vi "swerveImmForAuto.vi"(8 "scalespeed":dbl, 9 "x2":dbl, 10 "y1":dbl, 11 "x1":dbl) -> ()   [LabVIEW 2020]
uses:
  <vilib>/Rock Robotics/WPI/ThirdParty/Sensors/navX/_TypeDefs/FRIC_navX_DeviceNumbersTypeDef.ctl
  <vilib>/Rock Robotics/WPI/ThirdParty/REV Robotics/REVLib/Typedef/Spark MAX Control Type.ctl
  <vilib>/Rock Robotics/WPI/ThirdParty/Phoenix-LabVIEW/CANCoder/Get/CTRE_Phoenix_CANcoder_GetSensorData.vi
  <vilib>/addons/control/pid/pid.llb/PID (DBL).vi
  <vilib>/addons/control/pid/NI_PID_pid.lvlib
panel:
  in  "dt (s)":dbl=-1.0 format="%.3f"
  in  "PID gains 2":T1={"proportional gain (Kc)"=0.004667, "integral time (Ti, min)"=0.0, "derivative time (Td, min)"=0.0} {"derivative time (Td, min)" format="%.10f"; "integral time (Ti, min)" format="%.10f"; "proportional gain (Kc)" format="%.10f"}
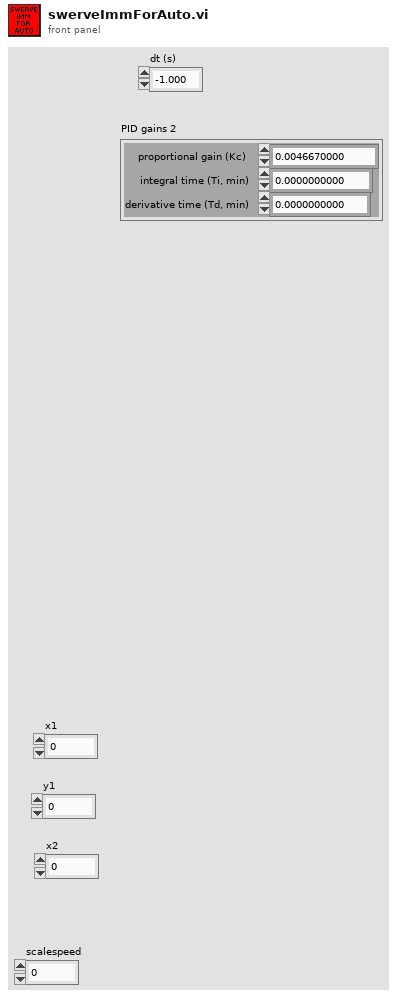
[diagram p1: front panel]
types:
  T1 = cluster{"proportional gain (Kc)":dbl, "integral time (Ti, min)":dbl, "derivative time (Td, min)":dbl}
  T2 = typedef "Spark MAX Control Type.ctl" = enum16{"Percent VBus", "Voltage", "Velocity", "Position", "Smart Motion", "Current", "Smart Velocity"}
  T3 = typedef "FRIC_navX_DeviceNumbersTypeDef.ctl" = enum16{"Dev0", "Dev1", "Dev2", "Dev3"}
  T4 = cluster{"Yaw":dbl, "Roll":dbl, "Pitch":dbl, "Heading":dbl, "Fused Heading":dbl}
  T5 = typedef "CTRE_Phoenix_CANcoder_DeviceRef.ctl" = cluster{"DeviceStatus":errorcluster, "Device Number":u8, "Handle":u64, "UsageFrame":u32, "Library Path":path}
  T6 = typedef "WPI_MotorControlDeviceRef.ctl" = cluster{"DeviceStatus":errorcluster, "Type":T7, "PWM":cluster{"PWM Channel":T8, "DeadBand":T9}, "CAN":cluster{"Device Number":u8, "SetOutput VI Ref":variant, "GetOutput VI Ref":variant, "Enable VI Ref":variant, "Disable VI Ref":variant, "Data":variant}, "Invert":bool, "DIO PWM":cluster{"PWM \"Enable\" Channel":T8, "DIOChannel":T10, "PWM Rate":dbl}}
  T7 = typedef "WPI_MotorControlType.ctl" = enum16{"PWM", "CAN", "DIO PWM"}
  T8 = typedef "FPGA_DIOPWMChannel.ctl" = enum8{"PWM 0", "PWM 1", "PWM 2", "PWM 3", "PWM 4", "PWM 5", "PWM 6", "PWM 7", "PWM 8", "PWM 9", "PWM MXP 0", "PWM MXP 1", "PWM MXP 2", "PWM MXP 3", "PWM MXP 4", "PWM MXP 5", "PWM MXP 6", "PWM MXP 7", "PWM MXP 8", "PWM MXP 9", "Invalid"}
  T9 = typedef "WPI_PWMDeadband.ctl" = cluster{"Name":string, "maxPositivePwm":i32, "minPositivePwm":i32, "centerPwm":i32, "maxNegativePwm":i32, "minNegativePwm":i32, "angularRange":u16}
  T10 = typedef "FPGA_DIOChannel.ctl" = enum8{"DIO 0", "DIO 1", "DIO 2", "DIO 3", "DIO 4", "DIO 5", "DIO 6", "DIO 7", "DIO 8", "DIO 9", "DIO MXP 0", "DIO MXP 1", "DIO MXP 2", "DIO MXP 3", "DIO MXP 4", "DIO MXP 5", "DIO MXP 6", "DIO MXP 7", "DIO MXP 8", "DIO MXP 9", "DIO MXP 10", "DIO MXP 11", "DIO MXP 12", "DIO MXP 13", "DIO MXP 14", "DIO MXP 15", "SPI Port CS1", "SPI Port CS2", "SPI Port CS3", "SPI Port MISO", "SPI Port MOSI", "Invalid"}
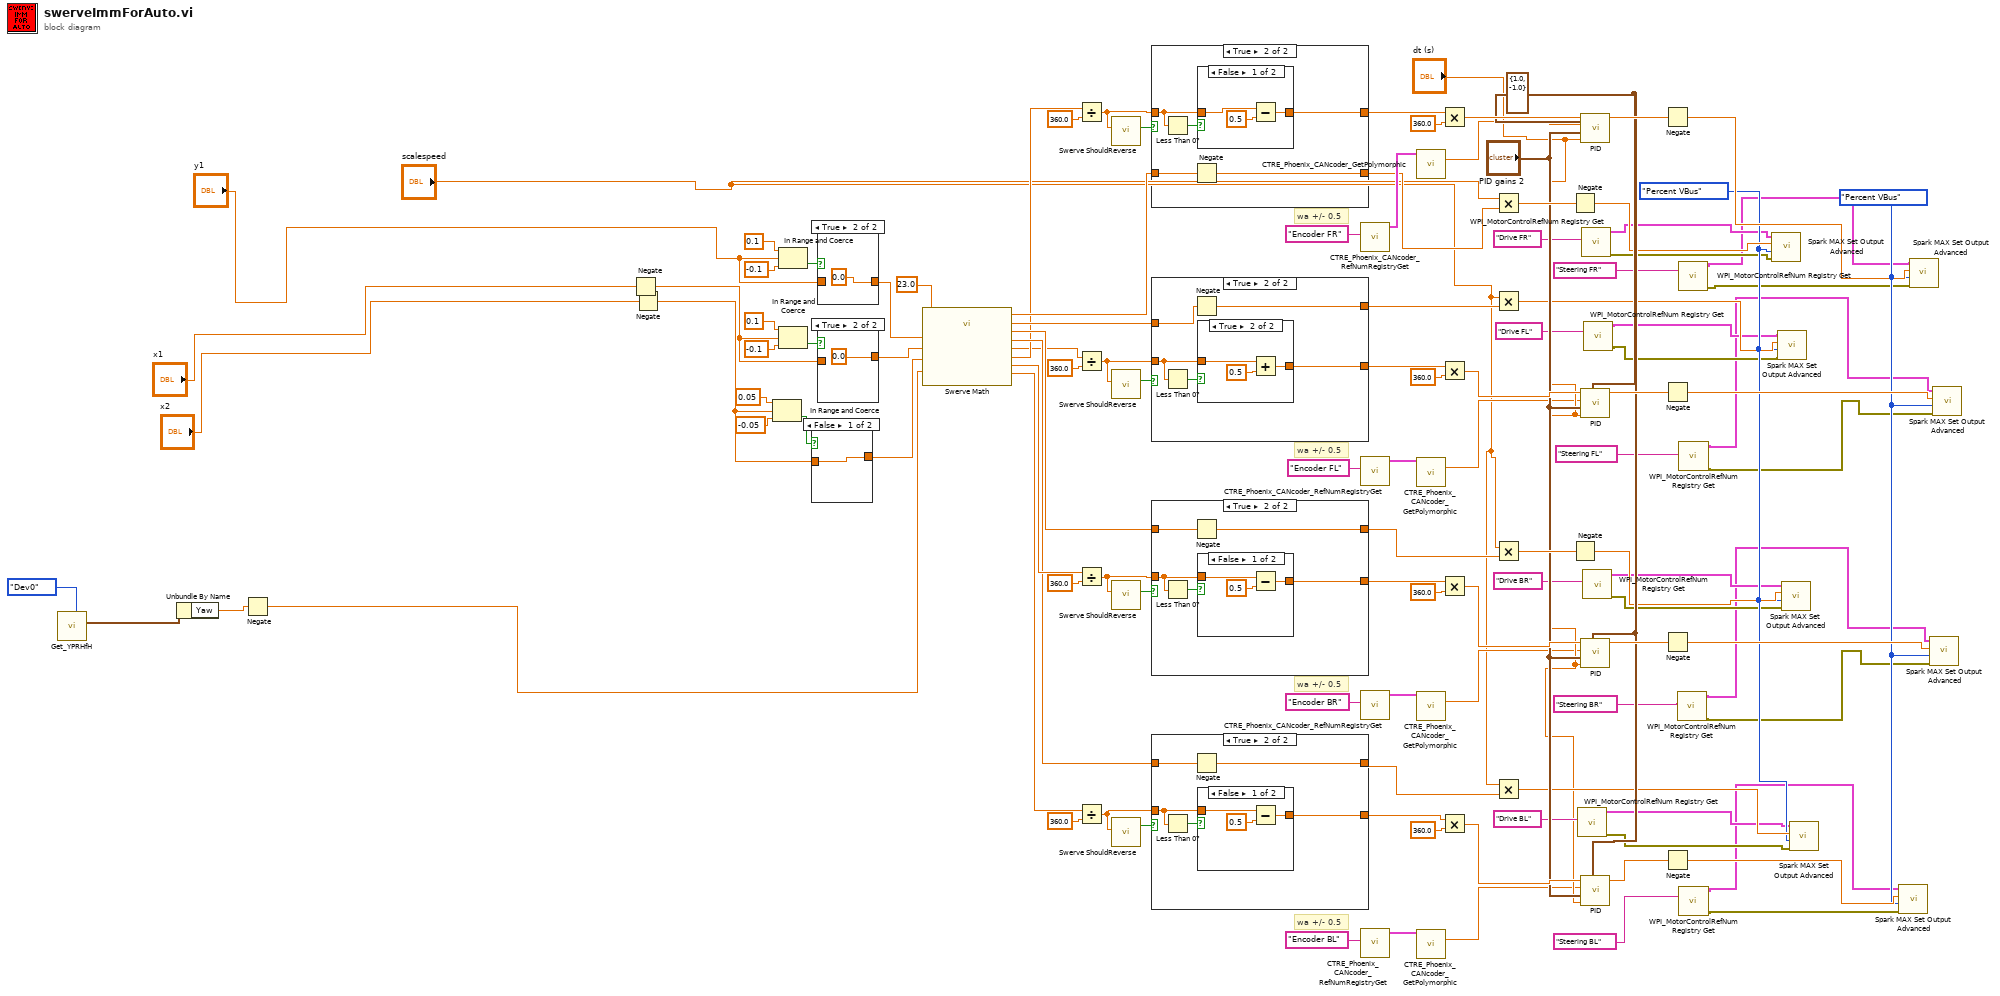
[diagram p0: block diagram]
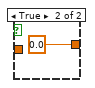
[diagram p2: hidden frame]
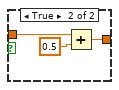
[diagram p4: hidden frame]
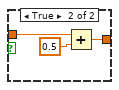
[diagram p6: hidden frame]
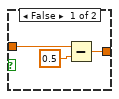
[diagram p8: hidden frame]
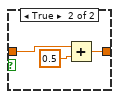
[diagram p10: hidden frame]
diagram:
  w43 = Spark_MAX_Control_Type."Percent VBus" ("Control Mode")
  w48 = Spark_MAX_Control_Type."Percent VBus" ("Control Mode")
  w53 = cluster{"output high":dbl, "output low":dbl} {"output high"=1.0, "output low"=-1.0} ("output range")
  w111 = 23.0 ("Trackwidth (W)")
  (unwired) FRIC_navX_DeviceNumbersTypeDef."Dev0" ("Device Number")
  # "wa +/- 0.5"
  # "wa +/- 0.5"
  # "wa +/- 0.5"
  # "wa +/- 0.5"
  n1 = call <vilib>:"Get_YPRHfH.vi"("Device Number"=FRIC_navX_DeviceNumbersTypeDef."Dev0") -> ("YRPHfH"=w113:T4)  [unwired: 10 in]
  n2 = Unbundle By Name(w113) -> ("Yaw"=w112:dbl)
  n3 = Negate(x=w112) -> (-x=w2:dbl)
  n4 = Negate(x="x1") -> (-x=w13:dbl)
  n5 = Negate(x="x2") -> (-x=w1:dbl)
  n6 = In Range and Coerce(upper limit=0.05, x=w1, lower limit=-0.05) -> (In Range?=w6:bool)  [unwired: 1 out]
  n7 = In Range and Coerce(upper limit=0.1, x="y1", lower limit=-0.1) -> (In Range?=w105:bool)  [unwired: 1 out]
  n8 = In Range and Coerce(upper limit=0.1, x=w13, lower limit=-0.1) -> (In Range?=w104:bool)  [unwired: 1 out]
  n9 = case shown="False" w6 {
    tunnel: [w115 0.0 ("upper limit")] -> w3
    tunnel: w1 -> [w115 _]
    frame False {
    }
    frame True {
    }
  }
  n10 = case shown="True" w105 {
    tunnel: [w117 0.0 ("upper limit")] -> w100
    tunnel: "y1" -> [w117 _]
    frame False {
    }
    frame True {
    }
  }
  n11 = case shown="True" w104 {
    tunnel: [w119 0.0 ("upper limit")] -> w101
    tunnel: w13 -> [w119 _]
    frame False {
    }
    frame True {
    }
  }
  n12 = call "Swerve Math.vi"("Trackwidth (W)"=w111, "Wheelbase (L)"=w111, "Y -FWD"=w100, "X1 STR"=w101, "X2 RCW"=w3, "Gyro Angle in degrees"=w2) -> ("wa3"=w57:dbl, "wa4"=w55:dbl, "ws1"=w60:dbl, "ws2"=w59:dbl, "ws3"=w58:dbl, "ws4"=w56:dbl, "wa2"=w12:dbl, "wa1"=w11:dbl)  [unwired: 2 in]
  n13 = Divide(x=w12, y=360.0) -> (x/y=w97:dbl)
  n14 = Divide(x=w11, y=360.0) -> (x/y=w86:dbl)
  n15 = Divide(x=w57, y=360.0) -> (x/y=w76:dbl)
  n16 = Divide(x=w55, y=360.0) -> (x/y=w65:dbl)
  n17 = call "Swerve ShouldReverse.vi"("wa in"=w97) -> ("shouldReverse out"=w98:bool)  [unwired: 10 in]
  n18 = call "Swerve ShouldReverse.vi"("wa in"=w86) -> ("shouldReverse out"=w87:bool)  [unwired: 10 in]
  n19 = call "Swerve ShouldReverse.vi"("wa in"=w76) -> ("shouldReverse out"=w77:bool)  [unwired: 10 in]
  n20 = call "Swerve ShouldReverse.vi"("wa in"=w65) -> ("shouldReverse out"=w66:bool)  [unwired: 10 in]
  n21 = case shown="True" w98 {
    tunnel: w60 -> [w122 w123]
    tunnel: w97 -> [w121 w126]
    tunnel: [w122 w124] -> w96
    tunnel: [w121 w125] -> w95
    frame False {
    }
    frame True {
      n22 = Less Than 0?(x=w126) -> (x < 0?=w127:bool)
      n23 = Negate(x=w123) -> (-x=w124:dbl)
      n24 = case shown="False" w127 {
        tunnel: w126 -> [w129 w132]
        tunnel: [w128 w131] -> w125
        frame False {
          n25 = Subtract(x=w129, y=0.5) -> (x-y=w128:dbl)
        }
        frame True {
          n26 = Add(x=w132, y=0.5) -> (x+y=w131:dbl)
        }
      }
    }
  }
  n27 = case shown="True" w87 {
    tunnel: w59 -> [w135 w136]
    tunnel: w86 -> [w134 w139]
    tunnel: [w135 w137] -> w85
    tunnel: [w134 w138] -> w84
    frame False {
    }
    frame True {
      n28 = Less Than 0?(x=w139) -> (x < 0?=w140:bool)
      n29 = Negate(x=w136) -> (-x=w137:dbl)
      n30 = case shown="True" w140 {
        tunnel: w139 -> [w142 w145]
        tunnel: [w141 w144] -> w138
        frame False {
          n31 = Subtract(x=w142, y=0.5) -> (x-y=w141:dbl)
        }
        frame True {
          n32 = Add(x=w145, y=0.5) -> (x+y=w144:dbl)
        }
      }
    }
  }
  n33 = case shown="True" w77 {
    tunnel: w58 -> [w148 w149]
    tunnel: w76 -> [w147 w152]
    tunnel: [w148 w150] -> w75
    tunnel: [w147 w151] -> w74
    frame False {
    }
    frame True {
      n34 = Less Than 0?(x=w152) -> (x < 0?=w153:bool)
      n35 = Negate(x=w149) -> (-x=w150:dbl)
      n36 = case shown="False" w153 {
        tunnel: w152 -> [w155 w158]
        tunnel: [w154 w157] -> w151
        frame False {
          n37 = Subtract(x=w155, y=0.5) -> (x-y=w154:dbl)
        }
        frame True {
          n38 = Add(x=w158, y=0.5) -> (x+y=w157:dbl)
        }
      }
    }
  }
  n39 = case shown="True" w66 {
    tunnel: w56 -> [w161 w162]
    tunnel: w65 -> [w160 w165]
    tunnel: [w161 w163] -> w64
    tunnel: [w160 w164] -> w63
    frame False {
    }
    frame True {
      n40 = Less Than 0?(x=w165) -> (x < 0?=w166:bool)
      n41 = Negate(x=w162) -> (-x=w163:dbl)
      n42 = case shown="False" w166 {
        tunnel: w165 -> [w168 w171]
        tunnel: [w167 w170] -> w164
        frame False {
          n43 = Subtract(x=w168, y=0.5) -> (x-y=w167:dbl)
        }
        frame True {
          n44 = Add(x=w171, y=0.5) -> (x+y=w170:dbl)
        }
      }
    }
  }
  n45 = call <vilib>:"CTRE_Phoenix_CANcoder_RefNumRegistryGet.vi"("refnum name"="Encoder FR") -> ("CTRE_CANcoder_DeviceRef"=w109:T5)  [unwired: 9 in, 1 out]
  n46 = call <vilib>:"CTRE_Phoenix_CANcoder_RefNumRegistryGet.vi"("refnum name"="Encoder FL") -> ("CTRE_CANcoder_DeviceRef"=w90:T5)  [unwired: 9 in, 1 out]
  n47 = call <vilib>:"CTRE_Phoenix_CANcoder_RefNumRegistryGet.vi"("refnum name"="Encoder BR") -> ("CTRE_CANcoder_DeviceRef"=w80:T5)  [unwired: 9 in, 1 out]
  n48 = call <vilib>:"CTRE_Phoenix_CANcoder_RefNumRegistryGet.vi"("refnum name"="Encoder BL") -> ("CTRE_CANcoder_DeviceRef"=w69:T5)  [unwired: 9 in, 1 out]
  n49 = call-poly <vilib>:"CTRE_Phoenix_CANcoder_GetPolymorphic.vi"("CTRE_CANcoder_DeviceRef"=w109) -> ("Position"=w15:dbl)  [unwired: 10 in, 4 out]
  n50 = call-poly <vilib>:"CTRE_Phoenix_CANcoder_GetPolymorphic.vi"("CTRE_CANcoder_DeviceRef"=w90) -> ("Position"=w16:dbl)  [unwired: 10 in, 4 out]
  n51 = call-poly <vilib>:"CTRE_Phoenix_CANcoder_GetPolymorphic.vi"("CTRE_CANcoder_DeviceRef"=w80) -> ("Position"=w17:dbl)  [unwired: 10 in, 4 out]
  n52 = call-poly <vilib>:"CTRE_Phoenix_CANcoder_GetPolymorphic.vi"("CTRE_CANcoder_DeviceRef"=w69) -> ("Position"=w14:dbl)  [unwired: 10 in, 4 out]
  n53 = Multiply(x=w95, y=360.0) -> (x*y=w94:dbl)
  n54 = Multiply(x=w84, y=360.0) -> (x*y=w83:dbl)
  n55 = Multiply(x=w74, y=360.0) -> (x*y=w73:dbl)
  n56 = Multiply(x=w63, y=360.0) -> (x*y=w62:dbl)
  n57 = Multiply(x="scalespeed", y=w96) -> (x*y=w92:dbl)
  n58 = Multiply(x="scalespeed", y=w85) -> (x*y=w46:dbl)
  n59 = Multiply(x="scalespeed", y=w75) -> (x*y=w71:dbl)
  n60 = Multiply(x="scalespeed", y=w64) -> (x*y=w44:dbl)
  n61 = Negate(x=w92) -> (-x=w47:dbl)
  n62 = Negate(x=w71) -> (-x=w45:dbl)
  n63 = call <vilib>:"WPI_MotorControlRefNum Registry Get.vi"("refnum name"="Drive BL") -> ("error out"=w23:errorcluster, "MotorControlDevRef"=w24:T6)  [unwired: 9 in]
  n64 = call-poly <vilib>:"PID.vi"("output range"=w53, "dt (s)"="dt (s)", "PID gains"="PID gains 2", "process variable"=w15, "setpoint"=w94) -> ("output"=w110:dbl)  [unwired: 5 in, 1 out]
  n65 = call-poly <vilib>:"PID.vi"("output range"=w53, "dt (s)"="dt (s)", "PID gains"="PID gains 2", "process variable"=w16, "setpoint"=w83) -> ("output"=w91:dbl)  [unwired: 5 in, 1 out]
  n66 = call-poly <vilib>:"PID.vi"("output range"=w53, "dt (s)"="dt (s)", "PID gains"="PID gains 2", "process variable"=w17, "setpoint"=w73) -> ("output"=w81:dbl)  [unwired: 5 in, 1 out]
  n67 = call-poly <vilib>:"PID.vi"("output range"=w53, "dt (s)"="dt (s)", "PID gains"="PID gains 2", "process variable"=w14, "setpoint"=w62) -> ("output"=w70:dbl)  [unwired: 5 in, 1 out]
  n68 = call <vilib>:"WPI_MotorControlRefNum Registry Get.vi"("refnum name"="Drive FR") -> ("error out"=w40:errorcluster, "MotorControlDevRef"=w41:T6)  [unwired: 9 in]
  n69 = call <vilib>:"WPI_MotorControlRefNum Registry Get.vi"("refnum name"="Drive BR") -> ("error out"=w28:errorcluster, "MotorControlDevRef"=w29:T6)  [unwired: 9 in]
  n70 = call <vilib>:"WPI_MotorControlRefNum Registry Get.vi"("refnum name"="Drive FL") -> ("error out"=w34:errorcluster, "MotorControlDevRef"=w35:T6)  [unwired: 9 in]
  n71 = Negate(x=w110) -> (-x=w52:dbl)
  n72 = Negate(x=w91) -> (-x=w51:dbl)
  n73 = Negate(x=w81) -> (-x=w50:dbl)
  n74 = Negate(x=w70) -> (-x=w49:dbl)
  n75 = call <vilib>:"WPI_MotorControlRefNum Registry Get.vi"("refnum name"="Steering BR") -> ("error out"=w26:errorcluster, "MotorControlDevRef"=w27:T6)  [unwired: 9 in]
  n76 = call <vilib>:"WPI_MotorControlRefNum Registry Get.vi"("refnum name"="Steering FR") -> ("error out"=w37:errorcluster, "MotorControlDevRef"=w38:T6)  [unwired: 9 in]
  n77 = call <vilib>:"WPI_MotorControlRefNum Registry Get.vi"("refnum name"="Steering FL") -> ("error out"=w31:errorcluster, "MotorControlDevRef"=w32:T6)  [unwired: 9 in]
  n78 = call <vilib>:"WPI_MotorControlRefNum Registry Get.vi"("refnum name"="Steering BL") -> ("error out"=w20:errorcluster, "MotorControlDevRef"=w21:T6)  [unwired: 9 in]
  n79 = call <vilib>:"Spark MAX Set Output Advanced.vi"("error in (no error)"=w40, "Control Mode"=w43, "Setpoint"=w47, "MotorControlDevRef"=w41) -> ()  [unwired: 6 in, 2 out]
  n80 = call <vilib>:"Spark MAX Set Output Advanced.vi"("error in (no error)"=w34, "Control Mode"=w43, "Setpoint"=w46, "MotorControlDevRef"=w35) -> ()  [unwired: 6 in, 2 out]
  n81 = call <vilib>:"Spark MAX Set Output Advanced.vi"("error in (no error)"=w28, "Control Mode"=w43, "Setpoint"=w45, "MotorControlDevRef"=w29) -> ()  [unwired: 6 in, 2 out]
  n82 = call <vilib>:"Spark MAX Set Output Advanced.vi"("error in (no error)"=w23, "Control Mode"=w43, "Setpoint"=w44, "MotorControlDevRef"=w24) -> ()  [unwired: 6 in, 2 out]
  n83 = call <vilib>:"Spark MAX Set Output Advanced.vi"("error in (no error)"=w20, "Control Mode"=w48, "Setpoint"=w49, "MotorControlDevRef"=w21) -> ()  [unwired: 6 in, 2 out]
  n84 = call <vilib>:"Spark MAX Set Output Advanced.vi"("error in (no error)"=w37, "Control Mode"=w48, "Setpoint"=w52, "MotorControlDevRef"=w38) -> ()  [unwired: 6 in, 2 out]
  n85 = call <vilib>:"Spark MAX Set Output Advanced.vi"("error in (no error)"=w26, "Control Mode"=w48, "Setpoint"=w50, "MotorControlDevRef"=w27) -> ()  [unwired: 6 in, 2 out]
  n86 = call <vilib>:"Spark MAX Set Output Advanced.vi"("error in (no error)"=w31, "Control Mode"=w48, "Setpoint"=w51, "MotorControlDevRef"=w32) -> ()  [unwired: 6 in, 2 out]
